vi "Fdx Stop.vi"   [LabVIEW 2020, in "AIM664LV.lvlib"]
uses:
  AIM664LV.lvlib
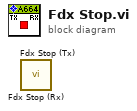
[diagram p0: block diagram]
diagram:
  n1 = call "Fdx Stop (Rx).vi"() -> ()  [unwired: 10 in, 2 out]
  n2 = call "Fdx Stop (Tx).vi"() -> ()  [unwired: 10 in, 2 out]
